vi "SDCP - Standard Message Frames Editor - Load Parameters From File.vi"(2 "error in (no error)":errorcluster, 3 "Parameter File Path":path=path "E:/Projects/System Diagnostics and Control Protocol/SDCP_LabVIEW/Parameter Files/test.param") -> (0 "error out":errorcluster, 1 "Output":T2(array[cluster]))   [LabVIEW 2020]
uses:
  Typedefs/SDCP - Standard Message Frames Editor - Parameter cluster.ctl
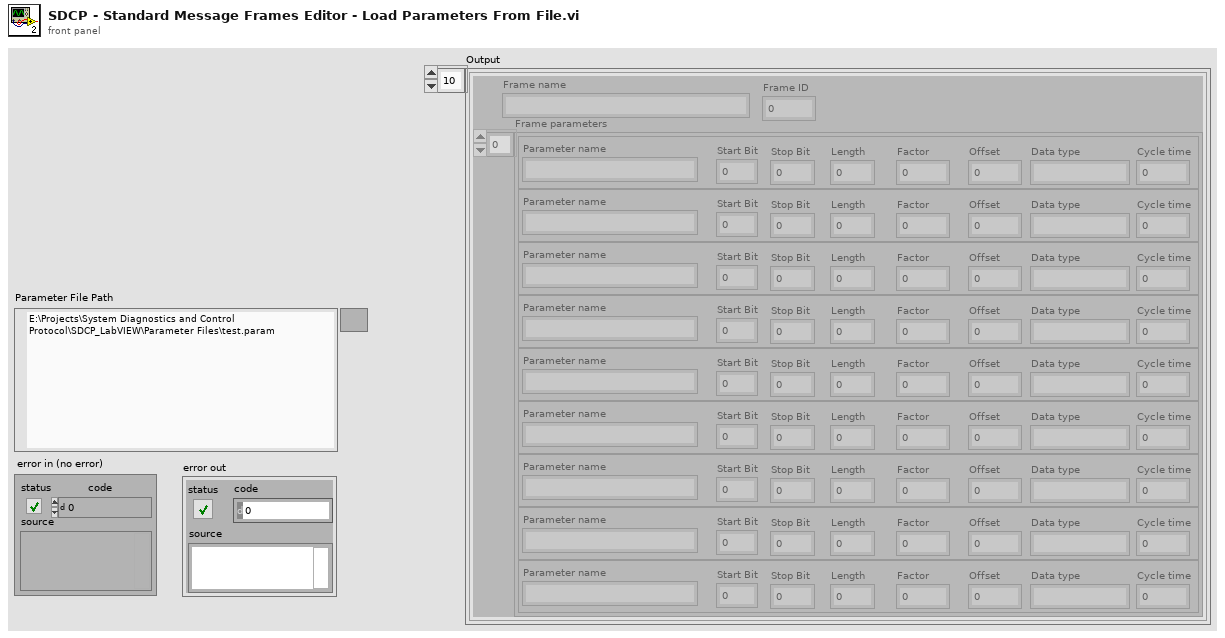
[diagram p1: front panel]
types:
  T1 = typedef "SDCP - Standard Message Frames Editor - Parameter cluster.ctl" = cluster{"Parameter name":string, "Start Bit":i32, "Stop Bit":i32, "Length":i32, "Factor":dbl, "Offset":dbl, "Data type":string, "Cycle time":dbl}
  T2 = cluster{"Frame name":string, "Frame ID":i32, "Frame parameters":T1[]}[]
  T3 = typedef "SDCP - SMF parameter descriptors.ctl" = cluster{"Frame name":string, "Frame ID":i32, "Data type":string, "Start Position":i32, "Length":i32, "Factor":dbl, "Offset":dbl, "Parameter name":string, "Value":string}
  T4 = cluster{"Frame name":string, "Frame ID":i32, "Frame parameters":T1[]}
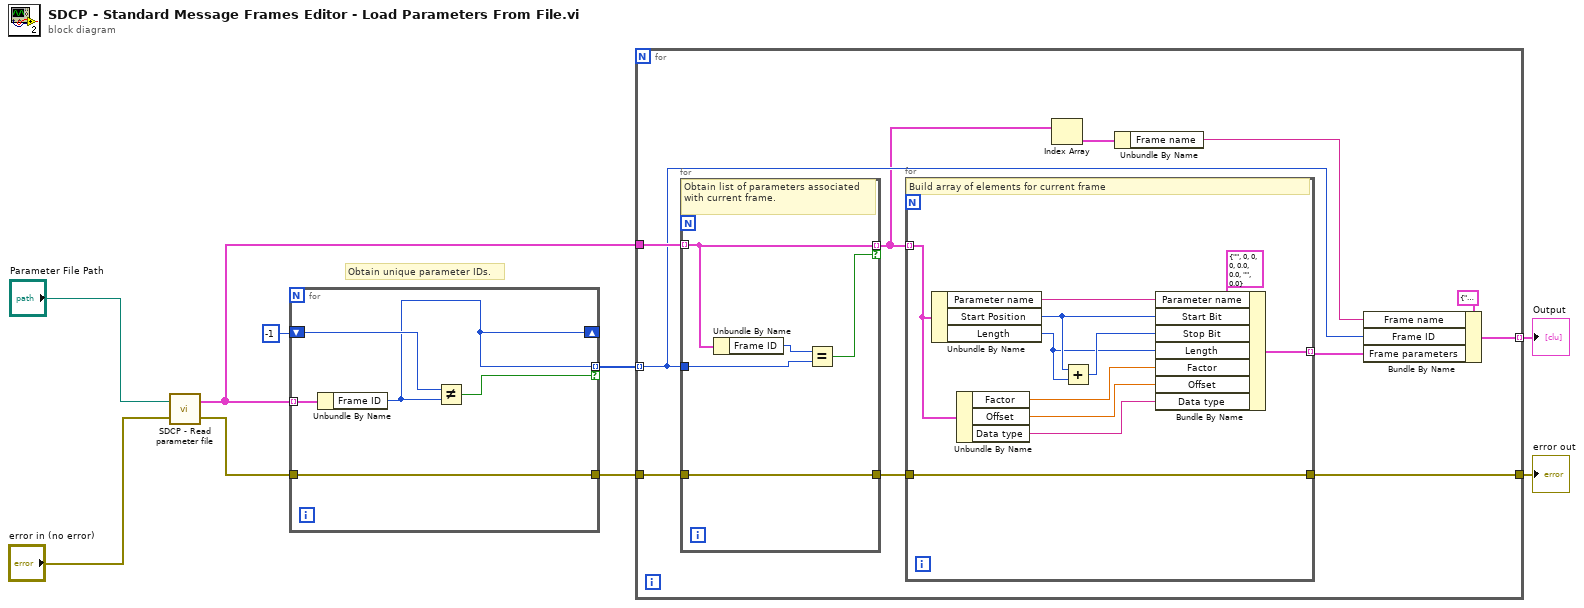
[diagram p0: block diagram]
diagram:
  # "Obtain unique parameter IDs."
  n1 = call "SDCP - Read parameter file.vi"("error in (no error)"="error in (no error)", "Parameter file path"="Parameter File Path") -> ("error out"=w7:errorcluster, "Parameter descriptors"=w3:T3[])
  n2 = for {
    tunnel: w7 -> [w10]
    tunnel: w3 -> [w14] mode=indexing
    shift-right: [w12] -> _
    shift-left: -1 -> [w13]
    tunnel: [w12] -> w4 mode=indexing if=w11
    tunnel: [w10] -> w5
    n3 = Unbundle By Name(w14) -> ("Frame ID"=w12:i32)
    n4 = Not Equal?(x=w13, y=w12) -> (x != y?=w11:bool)
  }
  n5 = for {
    tunnel: w5 -> [w25]
    tunnel: w4 -> [w20] mode=indexing
    tunnel: w3 -> [w24]
    tunnel: [w16] -> w1 mode=indexing
    tunnel: [w15] -> w2
    n6 = for {
      tunnel: w25 -> [w37]
      tunnel: w24 -> [w39] mode=indexing
      tunnel: w20 -> [w40]
      tunnel: [w39] -> w19 mode=indexing if=w38
      tunnel: [w37] -> w23
      # "Obtain list of parameters associated with current frame."
      n7 = Unbundle By Name(w39) -> ("Frame ID"=w41:i32)
      n8 = Equal?(x=w41, y=w40) -> (x = y?=w38:bool)
    }
    n9 = for {
      tunnel: w23 -> [w27]
      tunnel: w19 -> [w31] mode=indexing
      tunnel: [w27] -> w15
      tunnel: [w26] -> w21 mode=indexing
      # "Build array of elements for current frame"
      n10 = Unbundle By Name(w31) -> ("Parameter name"=w35:string, "Start Position"=w34:i32, "Length"=w32:i32)
      n11 = Unbundle By Name(w31) -> ("Factor"=w30:dbl, "Offset"=w29:dbl, "Data type"=w28:string)
      n12 = Add(x=w34, y=w32) -> (x+y=w33:i32)
      n13 = Bundle By Name(cluster=T1 {"Parameter name"="", "Start Bit"=0, "Stop Bit"=0, "Length"=0, "Factor"=0.0, "Offset"=0.0, "Data type"="", "Cycle time"=0.0}, "Parameter name"=w35, "Start Bit"=w34, "Stop Bit"=w33, "Length"=w32, "Factor"=w30, "Offset"=w29, "Data type"=w28) -> (w26:T1)
    }
    n14 = Index Array(array=w19) -> (element=w18:T3)  [unwired: 1 in]
    n15 = Unbundle By Name(w18) -> ("Frame name"=w17:string)
    n16 = Bundle By Name(cluster=T4 {"Frame name"="", "Frame ID"=0, "Frame parameters"=[]}, "Frame name"=w17, "Frame ID"=w20, "Frame parameters"=w21) -> (w16:T4)
  }
  "error out" <- w2
  "Output" <- w1
